vi "Test.vi"() -> ()   [LabVIEW 2018]
uses:
  LibTiePie.lvlib
panel:
  out "error out":errorcluster
  out "OscilloscopeCluster":T1
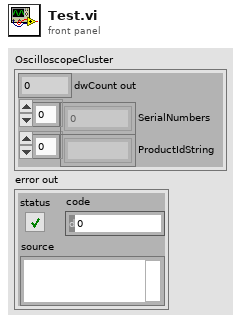
[diagram p1: front panel]
types:
  T1 = cluster{"dwCount out":u32, "SerialNumbers":u32[], "ProductIdString":string[]}
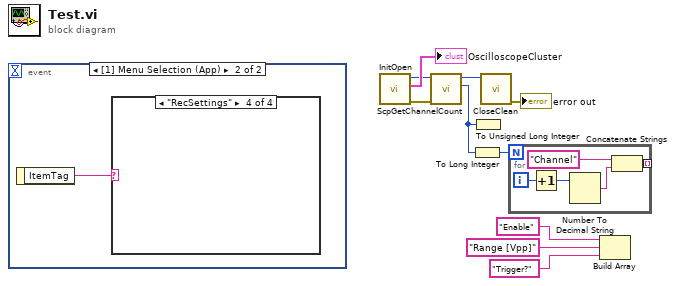
[diagram p0: block diagram]
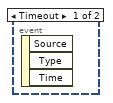
[diagram p2: hidden frame]
diagram:
  n1 = event shown="[1] Menu Selection (App)" {
    selector: _ -> [_ _]
    dyn-events: _ -> [_ _]
    timeout: _ -> [_ _]
    event Timeout {
      n2 = event-data() -> ()  [unwired: 1 in, 3 out]
    }
    event Menu Selection (App) {
      n3 = event-data() -> ("ItemTag"=w11:string)  [unwired: 1 in]
      n4 = case shown="\"RecSettings\"" w11 {
        frame "SaveAs" {
        }
        frame "ChSettings" {
        }
        frame "LogSettings" {
        }
        frame "RecSettings" {
        }
      }
    }
  }
  n5 = call "InitOpen.vi"() -> ("error out"=w7:errorcluster, "OscilloscopeCluster"=→"OscilloscopeCluster":T1, "hDevice"=w8:u32)  [unwired: 8 in]
  n6 = call "ScpGetChannelCount.vi"("error in (no error)"=w7, "hDevice in"=w8) -> ("wCh"=w4:u16, "hDevice out"=w6:u32)  [unwired: 7 in, 1 out]
  n7 = To Long Integer(number=w4) -> (32bit integer=w5:i32)
  n8 = To Unsigned Long Integer(number=w4) -> ()  [unwired: 1 out]
  n9 = call "CloseClean.vi"("hHandle"=w6) -> ("error out"=→"error out":errorcluster)  [unwired: 10 in]
  n10 = for {
    N: w5 -> [_]
    tunnel: [w12] -> _ mode=indexing
    i -> [w16]
    n11 = Increment(x=w16) -> (x+1=w14:i32)
    n12 = Number To Decimal String(number=w14) -> (decimal integer string=w13:string)  [unwired: 1 in]
    n13 = Concatenate Strings("Channel", w13) -> (w12:string)
  }
  n14 = Build Array("Enable", "Range [Vpp]", "Trigger?") -> ()  [unwired: 1 out]
